vi "Search.vi"(8 "error in":errorcluster, 11 "Driver path":path) -> (0 "error out":errorcluster, 3 "Enrolled ID":i32)   [LabVIEW 2020, in "r307-python-labview-driver.lvlib"]
uses:
  r307-python-labview-driver.lvlib
  <vilib>/Utility/error.llb/whitespace.ctl
panel:
  out "Found":bool
  out "command line":string="cmc /c python \"%s\" ENROLL"
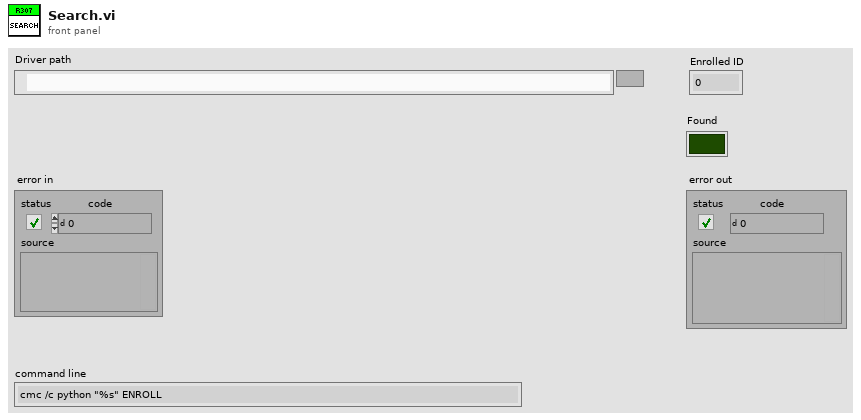
[diagram p1: front panel]
types:
  T1 = typedef "whitespace.ctl" = u16
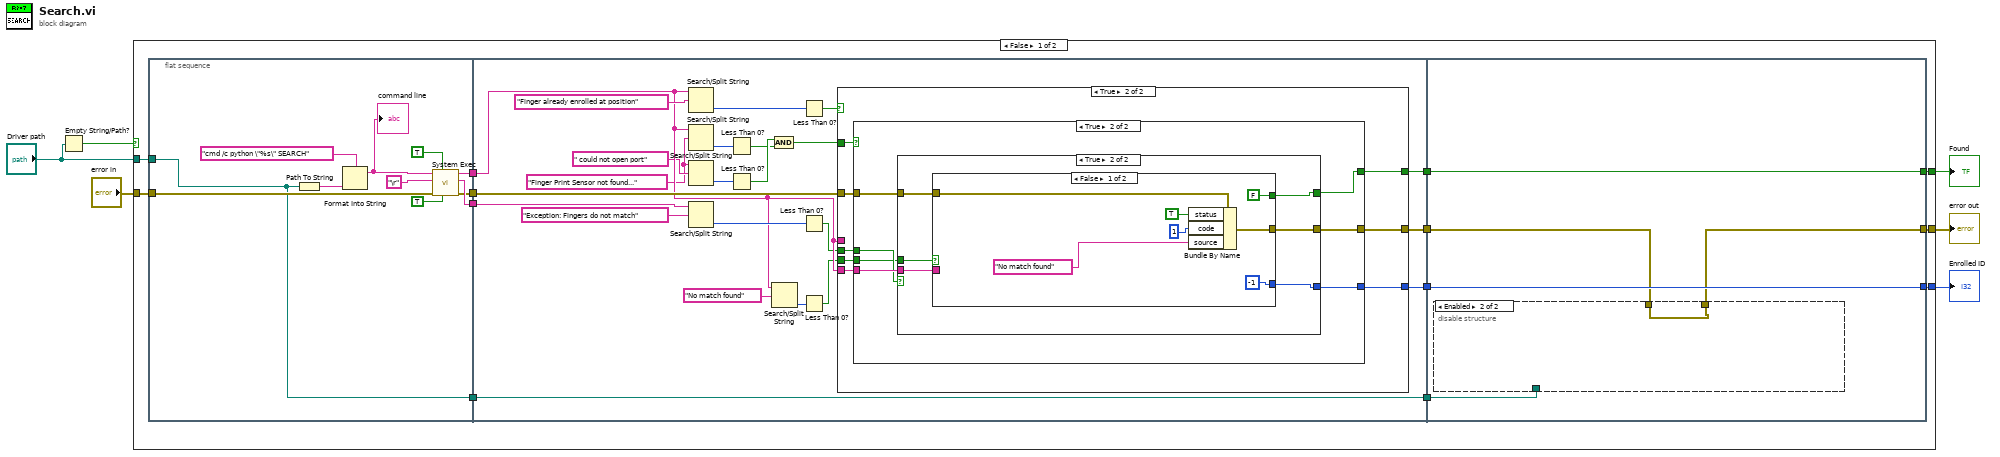
[diagram p0: block diagram]
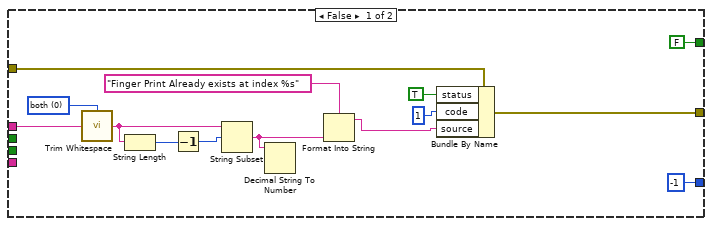
[diagram p2: hidden frame]
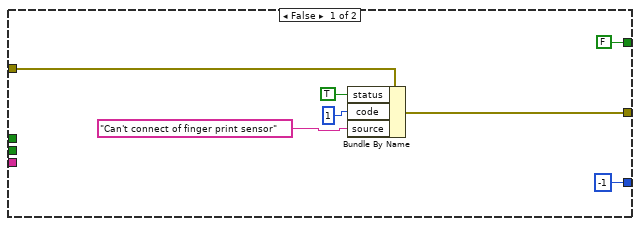
[diagram p3: hidden frame]
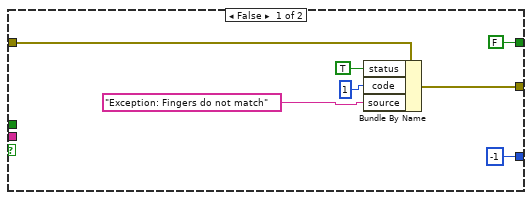
[diagram p4: hidden frame]
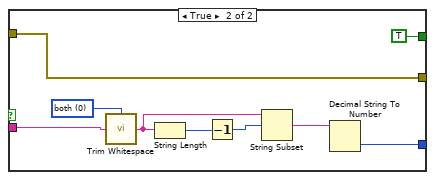
[diagram p5: hidden frame]
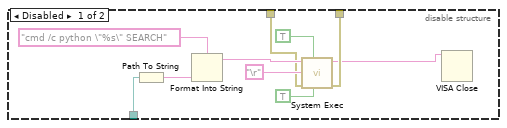
[diagram p6: hidden frame]
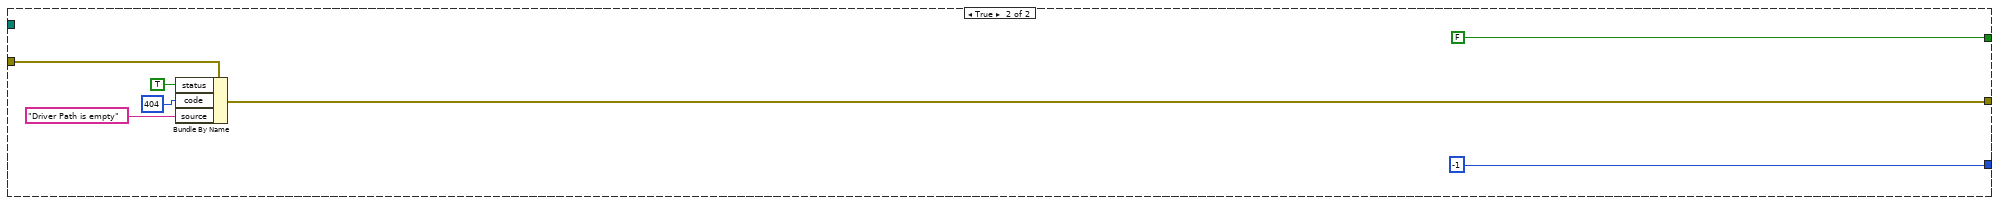
[diagram p7: hidden frame]
diagram:
  n1 = Empty String/Path?(string/path="Driver path") -> (empty?=w2:bool)
  n2 = case shown="False" w2 {
    tunnel: "Driver path" -> [w16 _]
    tunnel: "error in" -> [w15 w140]
    tunnel: [w14 w136] -> w5
    tunnel: [w13 -1 ("Enrolled ID")] -> w4
    tunnel: [w12 FALSE ("Found")] -> w3
    frame False {
      n3 = flat-sequence {
        tunnel: w16 -> [w20]
        tunnel: w15 -> [w22]
        tunnel: [w25] -> w19
        tunnel: [w21] -> w18
        tunnel: [w24] -> w17
        tunnel: [w20] -> w7
        tunnel: w19 -> [w52]
        tunnel: w18 -> [w51]
        tunnel: w17 -> [w41]
        tunnel: [w47] -> w11
        tunnel: [w45] -> w10
        tunnel: [w39] -> w9
        tunnel: [w32] -> w8
        tunnel: w7 -> [w32]
        tunnel: [w122] -> w12
        tunnel: [w123] -> w13
        tunnel: [w119] -> w14
        tunnel: w11 -> [w120]
        tunnel: w10 -> [w123]
        tunnel: w9 -> [w122]
        tunnel: w8 -> [w121]
        frame #0 {
          n4 = Path To String(path=w20) -> (string=w27:string)
          n5 = Format Into String(format string="cmd /c python \"%s\" SEARCH" ("command line"), w27) -> (resulting string=w28:string)  [unwired: 2 in, 1 out]
          "command line" <- w28
          n6 = call <vilib>:"System Exec.vi"("run minimized? (F)"=TRUE, "wait until completion? (T)"=TRUE, "error in (no error)"=w22, "standard input"="\r", "command line"=w28) -> ("error out"=w21:errorcluster, "standard error"=w25:string, "standard output"=w24:string)  [unwired: 3 in, 1 out]
        }
        frame #1 {
          w33 = "Finger Print Sensor not found..." ("search string/char (-)")
          n7 = Search/Split String(string=w41, search string/char (-)="Finger already enrolled at position") -> (offset of match=w43:i32)  [unwired: 1 in, 2 out]
          n8 = Search/Split String(string=w41, search string/char (-)=w33) -> (offset of match=w50:i32)  [unwired: 1 in, 2 out]
          n9 = Search/Split String(string=w33, search string/char (-)=" could not open port") -> (offset of match=w38:i32)  [unwired: 1 in, 2 out]
          n10 = Search/Split String(string=w52, search string/char (-)="Exception: Fingers do not match") -> (offset of match=w53:i32)  [unwired: 1 in, 2 out]
          n11 = Less Than 0?(x=w50) -> (x < 0?=w36:bool)
          n12 = Less Than 0?(x=w38) -> (x < 0?=w37:bool)
          n13 = And(x=w37, y=w36) -> (x .and. y?=w35:bool)
          n14 = Search/Split String(string=w41, search string/char (-)="No match found" ("string")) -> (offset of match=w49:i32)  [unwired: 1 in, 2 out]
          n15 = Less Than 0?(x=w43) -> (x < 0?=w42:bool)
          n16 = Less Than 0?(x=w53) -> (x < 0?=w40:bool)
          n17 = Less Than 0?(x=w49) -> (x < 0?=w31:bool)
          n18 = case shown="True" w42 {
            tunnel: w51 -> [w65 w75]
            tunnel: w35 -> [_ w74]
            tunnel: [w62 w73] -> w47
            tunnel: w41 -> [_ w72]
            tunnel: [-1 ("Enrolled ID") w71] -> w45
            tunnel: w41 -> [w58 _]
            tunnel: w40 -> [_ w70]
            tunnel: w31 -> [_ w69]
            tunnel: [FALSE ("Found") w68] -> w39
            frame False {
              w59 = T1 0 items=["both", "start of string", "end of string"] ("location (both)")
              n19 = call <vilib>:"Trim Whitespace.vi"("string"=w58, "location (both)"=w59) -> ("trimmed string"=w55:string)
              n20 = String Length(string=w55) -> (length=w57:i32)
              n21 = Decrement(x=w57) -> (x-1=w56:i32)
              n22 = String Subset(string=w55, offset (0)=w56) -> (substring=w60:string)  [unwired: 1 in]
              n23 = Decimal String To Number(string=w60) -> ()  [unwired: 2 in, 2 out]
              n24 = Format Into String(format string="Finger Print Already exists at index %s" ("source"), w60) -> (resulting string=w63:string)  [unwired: 2 in, 1 out]
              n25 = Bundle By Name(cluster=w65, "status"=TRUE, "code"=1, "source"=w63) -> (w62:errorcluster)
            }
            frame True {
              n26 = case shown="True" w74 {
                tunnel: w75 -> [w79 w89]
                tunnel: w72 -> [_ w87]
                tunnel: [w78 w88] -> w73
                tunnel: [-1 ("Enrolled ID") w86] -> w71
                tunnel: w70 -> [_ w85]
                tunnel: w69 -> [_ w84]
                tunnel: [FALSE ("Found") w83] -> w68
                frame False {
                  n27 = Bundle By Name(cluster=w79, "status"=TRUE, "code"=1, "source"="Can't connect of finger print sensor" ("search string/char (-)")) -> (w78:errorcluster)
                }
                frame True {
                  n28 = case shown="True" w85 {
                    tunnel: w89 -> [w96 w99]
                    tunnel: [w93 w98] -> w88
                    tunnel: w87 -> [_ w102]
                    tunnel: [-1 ("Enrolled ID") w101] -> w86
                    tunnel: w84 -> [_ w100]
                    tunnel: [FALSE ("Found") w97] -> w83
                    frame False {
                      n29 = Bundle By Name(cluster=w96, "status"=TRUE, "code"=1, "source"="Exception: Fingers do not match" ("search string/char (-)")) -> (w93:errorcluster)
                    }
                    frame True {
                      n30 = case shown="False" w100 {
                        tunnel: w102 -> [_ w112]
                        tunnel: [-1 w117] -> w101
                        tunnel: w99 -> [w106 w114]
                        tunnel: [w105 w114] -> w98
                        tunnel: [FALSE ("Found") TRUE ("Found")] -> w97
                        frame False {
                          n31 = Bundle By Name(cluster=w106, "status"=TRUE, "code"=1, "source"="No match found" ("string")) -> (w105:errorcluster)
                        }
                        frame True {
                          w113 = T1 0 items=["both", "start of string", "end of string"] ("location (both)")
                          n32 = call <vilib>:"Trim Whitespace.vi"("string"=w112, "location (both)"=w113) -> ("trimmed string"=w111:string)
                          n33 = String Length(string=w111) -> (length=w116:i32)
                          n34 = Decrement(x=w116) -> (x-1=w115:i32)
                          n35 = String Subset(string=w111, offset (0)=w115) -> (substring=w118:string)  [unwired: 1 in]
                          n36 = Decimal String To Number(string=w118) -> (number=w117:i32)  [unwired: 2 in, 1 out]
                        }
                      }
                    }
                  }
                }
              }
            }
          }
        }
        frame #2 {
          n37 = disable-structure shown="Enabled" {
            disable-tunnel: w121 -> [w127 _]
            disable-tunnel: w120 -> [w126 w134]
            disable-tunnel: [w125 w134] -> w119
            frame Disabled {
              n38 = Path To String(path=w127) -> (string=w132:string)
              n39 = Format Into String(format string="cmd /c python \"%s\" SEARCH" ("command line"), w132) -> (resulting string=w133:string)  [unwired: 2 in, 1 out]
              n40 = call <vilib>:"System Exec.vi"("run minimized? (F)"=TRUE, "wait until completion? (T)"=TRUE, "error in (no error)"=w126, "standard input"="\r", "command line"=w133) -> ("error out"=w125:errorcluster, "standard output"=w124:string)  [unwired: 3 in, 2 out]
              n41 = VISA Close(VISA resource name=w124) -> ()  [unwired: 1 in, 1 out]
            }
            frame Enabled {
            }
          }
        }
      }
    }
    frame True {
      n42 = Bundle By Name(cluster=w140, "status"=TRUE, "code"=404, "source"="Driver Path is empty") -> (w136:errorcluster)
    }
  }
  "error out" <- w5
  "Enrolled ID" <- w4
  "Found" <- w3
